vi "HM8118 - Read All Measurements.vi"(8 "error in (no error)":errorcluster, 11 "VISA resource name":refnum<visa-resource-name>) -> (0 "error out":errorcluster, 1 "Secondary":dbl, 2 "Primary":dbl, 3 "VISA resource name out":refnum<visa-resource-name>, 5 "Number of Bins":dbl)   [LabVIEW 2017]
doc: "Reads and returns the primary and secondary measurements from the instrument. Use this VI when you want to take multiple measurements using an immediate trigger. Use the low-level VIs for other triggering options."
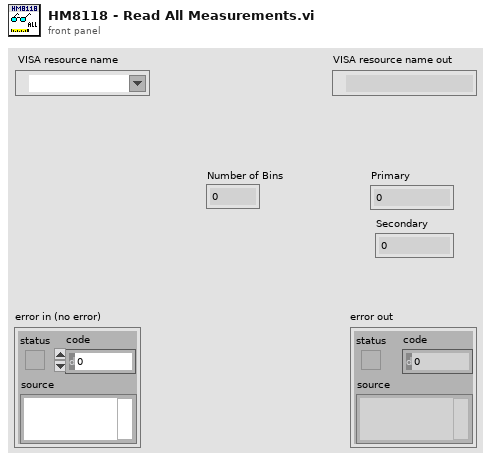
[diagram p1: front panel]
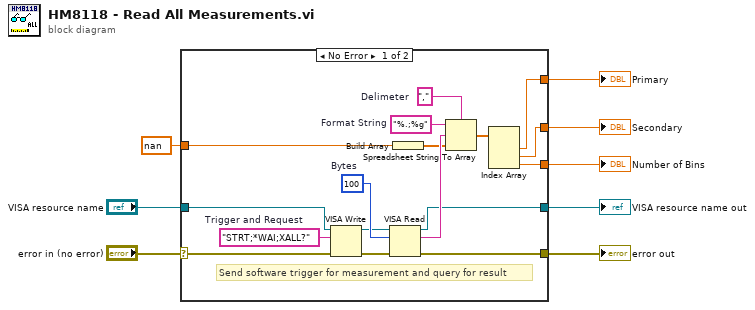
[diagram p0: block diagram]
diagram:
  n1 = case shown="No Error" "error in (no error)" {
    selector: "error in (no error)" -> [w9 w28]
    tunnel: "VISA resource name" -> [w24 w27]
    tunnel: nan -> [w20 w26]
    tunnel: [w16 w26] -> w6
    tunnel: [w15 w26] -> w5
    tunnel: [w14 w26] -> w4
    tunnel: [w12 w28] -> w3
    tunnel: [w11 w27] -> w2
    frame No Error {
      w18 = "STRT;*WAI;XALL?"  # Trigger and Request
      w21 = ","  # Delimeter
      w22 = "%.;%g"  # Format String
      w25 = u32 100  # Bytes
      # "Send software trigger for measurement and query for result"
      n2 = VISA Write(VISA resource name=w24, write buffer=w18, error in (no error)=w9) -> (VISA resource name out=w13:refnum<visa-resource-name>, error out=w10:errorcluster)  [unwired: 1 out]
      n3 = VISA Read(VISA resource name=w13, byte count=w25, error in (no error)=w10) -> (VISA resource name out=w11:refnum<visa-resource-name>, read buffer=w23:string, error out=w12:errorcluster)  [unwired: 1 out]
      n4 = Build Array(w20) -> (w19:dbl[])
      n5 = Spreadsheet String To Array(delimiter (Tab)=w21, format string=w22, spreadsheet string=w23, array type (2D Dbl)=w19) -> (array=w17:dbl[])
      n6 = Index Array(array=w17) -> (element #1=w16:dbl, element #2=w15:dbl, element #3=w14:dbl)  [unwired: 3 in]
    }
    frame Error {
    }
  }
  "error out" <- w3
  "VISA resource name out" <- w2
  "Primary" <- w6
  "Secondary" <- w5
  "Number of Bins" <- w4
